vi "dfd_Get VI Description.vi"(11 "filter info":T1={"L"=13, "M"=1, "filter structure"="CIC", "input fxp type"={"Signed"=TRUE, "Word Length"=16, "Integer Word Length"=1}, "output fxp type"={"Signed"=TRUE, "Word Length"=16, "Integer Word Length"=2}, "output rounding mode"=enum."Truncate", "number of channels"=1, "algorithm"="DA", "estimated resouces"="LUT: 1000", "output overflow mode"=enum."Wrap", "throughput"=1.0, "gain processing"=1, "Inside SCTL?"=FALSE, "FIFO Wrapper ?"=FALSE} {"gain processing" items=["On Target", "On Host"]}) -> (3 "VI description":string)   [LabVIEW 2017, in "NI_DigFilterLicensed.lvlib"]
uses:
  <vilib>/addons/Digital Filter Design/NI_DigFilterLicensed.lvlib
  <vilib>/addons/Digital Filter Design/_Objects.llb/DFD Filter Info.ctl
  <vilib>/fxp/LVFixedPointRepBitsTypeDef.ctl
  <vilib>/fxp/LVFixedPointQuantizationPolicyTypeDef.ctl
  <vilib>/fxp/LVFixedPointOverflowPolicyTypeDef.ctl
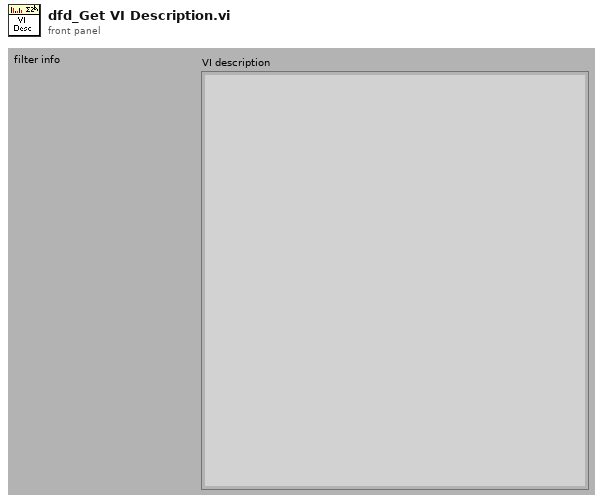
[diagram p1: front panel]
types:
  T1 = typedef "DFD Filter Info.ctl" = cluster{"L":i32, "M":i32, "filter structure":string, "input fxp type":T2, "output fxp type":T2, "output rounding mode":T3, "number of channels":i32, "algorithm":string, "estimated resouces":string, "output overflow mode":T4, "throughput":dbl, "gain processing":u16, "Inside SCTL?":bool, "FIFO Wrapper ?":bool}
  T2 = typedef "LVFixedPointRepBitsTypeDef.ctl" = cluster{"Signed":bool, "Word Length":u32, "Integer Word Length":i32}
  T3 = typedef "LVFixedPointQuantizationPolicyTypeDef.ctl" = enum32{"Truncate", "Round-Half-Up (Asymmetric)", "Round-Half-Even"}
  T4 = typedef "LVFixedPointOverflowPolicyTypeDef.ctl" = enum32{"Wrap", "Saturate"}
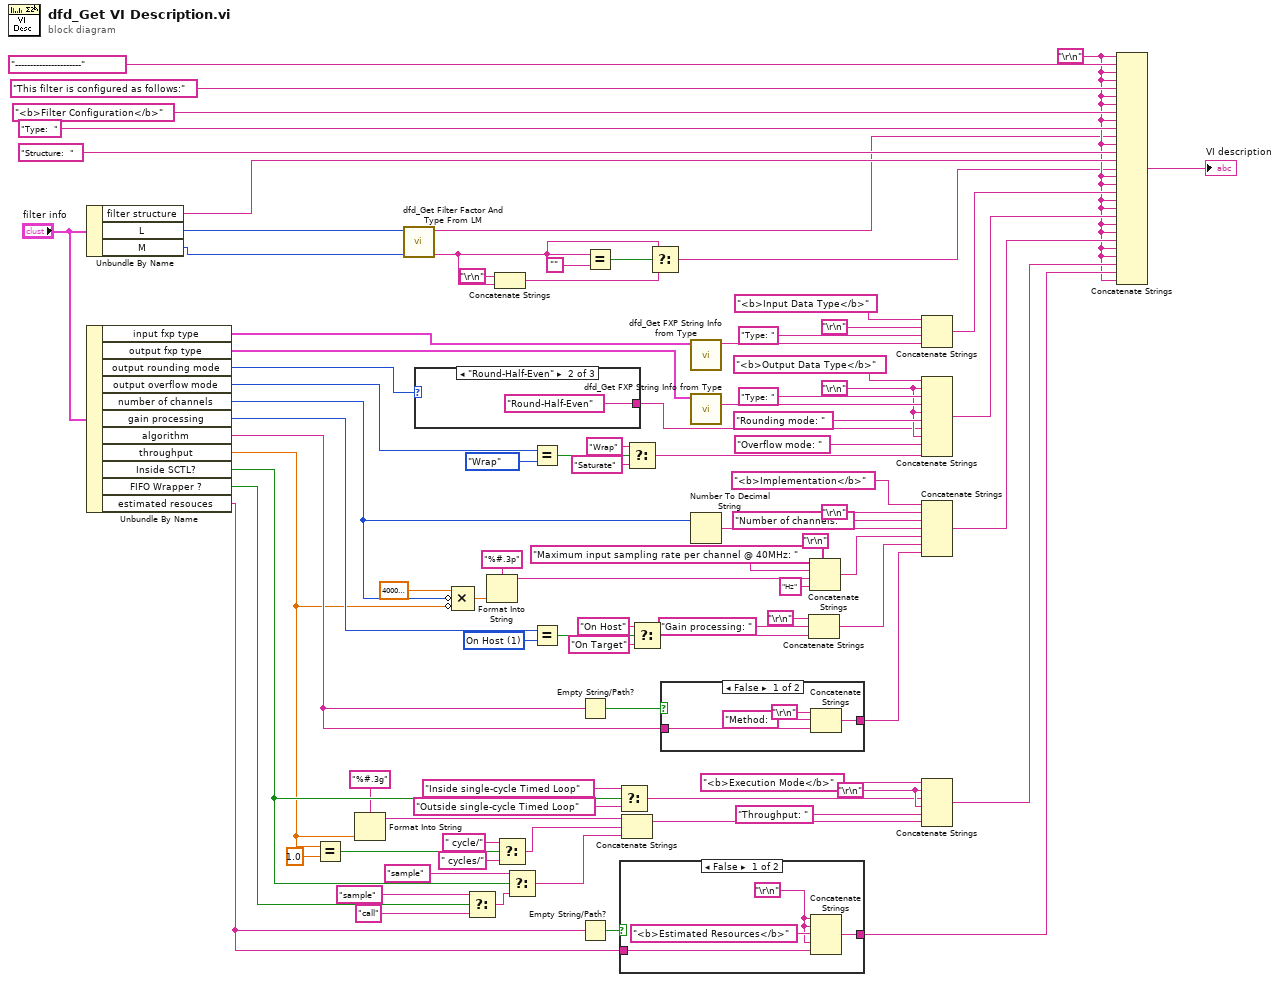
[diagram p0: block diagram]
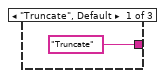
[diagram p2: hidden frame]
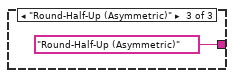
[diagram p3: hidden frame]
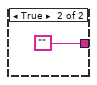
[diagram p4: hidden frame]
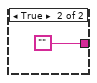
[diagram p5: hidden frame]
diagram:
  w49 = "\r\n"
  w54 = u16 1 items=["On Target", "On Host"] ("gain processing")
  w71 = "\r\n"
  w32 = "\r\n"
  n1 = Unbundle By Name("filter info") -> ("filter structure"=w87:string, "L"=w31:i32, "M"=w30:i32)
  n2 = Unbundle By Name("filter info") -> ("input fxp type"=w86:T2, "output fxp type"=w81:T2, "output rounding mode"=w41:T3, "output overflow mode"=w60:T4, "number of channels"=w13:i32, "gain processing"=w53:u16, "algorithm"=w67:string, "throughput"=w12:dbl, "Inside SCTL?"=w48:bool, "FIFO Wrapper ?"=w21:bool, "estimated resouces"=w22:string)
  n3 = Equal?(x=w12, y=1.0) -> (x = y?=w38:bool)
  n4 = Format Into String(format string="%#.3g", w12) -> (resulting string=w16:string)  [unwired: 2 in, 1 out]
  n5 = call <vilib>:"dfd_Get Filter Factor And Type From LM.vi"("M"=w30, "L"=w31) -> ("Factor"=w25:string, "Type"=w29:string)  [unwired: 8 out]
  n6 = case shown="\"Round-Half-Even\"" w41 {
    tunnel: ["Truncate" "Round-Half-Even" "Round-Half-Up (Asymmetric)"] -> w40
    frame "Truncate", Default {
    }
    frame "Round-Half-Even" {
    }
    frame "Round-Half-Up (Asymmetric)" {
    }
  }
  n7 = Compound Arithmetic op=MULTIPLY(40000000.0, invert w13, invert w12) -> (w9:dbl)
  n8 = Select(t="sample" ("string"), s=w21, f="call" ("string")) -> (s? t:f=w18:string)
  n9 = Format Into String(format string="%#.3p", w9) -> (resulting string=w7:string)  [unwired: 2 in, 1 out]
  n10 = Concatenate Strings("\r\n", w25) -> (w23:string)
  n11 = Select(t=" cycle/" ("string"), s=w38, f=" cycles/" ("string")) -> (s? t:f=w34:string)
  n12 = Select(t="sample" ("string"), s=w48, f=w18) -> (s? t:f=w35:string)
  n13 = Equal?(x=w60, y=LVFixedPointOverflowPolicyTypeDef."Wrap" ("output overflow mode")) -> (x = y?=w62:bool)
  n14 = Equal?(x=w53, y=w54) -> (x = y?=w57:bool)
  n15 = Empty String/Path?(string/path=w67) -> (empty?=w68:bool)
  n16 = Empty String/Path?(string/path=w22) -> (empty?=w66:bool)
  n17 = Equal?(x=w25, y="") -> (x = y?=w27:bool)
  n18 = Select(t="Inside single-cycle Timed Loop" ("string"), s=w48, f="Outside single-cycle Timed Loop" ("string")) -> (s? t:f=w46:string)
  n19 = case shown="False" w66 {
    tunnel: w22 -> [w98 _]
    tunnel: [w99 ""] -> w43
    frame False {
      w96 = "\r\n"
      n20 = Concatenate Strings(w96, w96, "<b>Estimated Resources</b>" ("string"), w96, w98) -> (w99:string)
    }
    frame True {
    }
  }
  n21 = Concatenate Strings(w16, w34, w35) -> (w58:string)
  n22 = Select(t="Wrap" ("string"), s=w62, f="Saturate") -> (s? t:f=w59:string)
  n23 = Select(t="On Host" ("string"), s=w57, f="On Target") -> (s? t:f=w4:string)
  n24 = Select(t=w25, s=w27, f=w23) -> (s? t:f=w26:string)
  n25 = case shown="False" w68 {
    tunnel: w67 -> [w104 _]
    tunnel: [w103 ""] -> w15
    frame False {
      n26 = Concatenate Strings("\r\n", "Method: " ("string"), w104) -> (w103:string)
    }
    frame True {
    }
  }
  n27 = call <vilib>:"dfd_Get FXP String Info from Type.vi"("fxp type"=w86) -> ("FXP Info String"=w83:string)  [unwired: 2 in, 8 out]
  n28 = call <vilib>:"dfd_Get FXP String Info from Type.vi"("fxp type"=w81) -> ("FXP Info String"=w74:string)  [unwired: 2 in, 8 out]
  n29 = Number To Decimal String(number=w13) -> (decimal integer string=w75:string)  [unwired: 1 out]
  n30 = Concatenate Strings("\r\n", "Gain processing: " ("string"), w4) -> (w1:string)
  n31 = Concatenate Strings("\r\n", "Maximum input sampling rate per channel @ 40MHz: " ("string"), w7, "Hz" ("string")) -> (w2:string)
  n32 = Concatenate Strings("<b>Input Data Type</b>", "\r\n", "Type: " ("string"), w83) -> (w84:string)
  n33 = Concatenate Strings("<b>Output Data Type</b>", w71, "Type: " ("string"), w74, w71, "Rounding mode: " ("string"), w40, w71, "Overflow mode: " ("string"), w59) -> (w79:string)
  n34 = Concatenate Strings("<b>Implementation</b>", "\r\n", "Number of channels: " ("string"), w75, w2, w1, w15) -> (w77:string)
  n35 = Concatenate Strings("<b>Execution Mode</b>", w49, w46, w49, "Throughput: " ("string"), w58) -> (w44:string)
  n36 = Concatenate Strings(w32, "----------------------", w32, w32, "This filter is configured as follows:", w32, w32, "<b>Filter Configuration</b>", w32, "Type:  ", w29, w32, "Structure:  ", w87, w26, w32, w32, w84, w32, w32, w79, w32, w32, w77, w32, w32, w44, w43, w32) -> (→"VI description":string)
